vi "SteuerungWaermepumpe.vi"() -> ()   [LabVIEW 2015]
uses:
  <vilib>/DAQmx/read.llb/DAQmx Read.vi
  <vilib>/DAQmx/read.llb/DAQmx Read (Analog 1D Wfm NChan NSamp).vi
  <vilib>/DAQmx/write.llb/DAQmx Write.vi
  <vilib>/DAQmx/write.llb/DAQmx Write (Analog 1D Wfm NChan 1Samp).vi
  <vilib>/MakerHub/LINX/Public/Peripherals/Digital/Digital Write N Chans.vi
  <vilib>/DAQmx/miscellaneous.llb/DAQmx Fill In Error Info.vi
  <vilib>/Utility/file.llb/Read Delimited Spreadsheet (DBL).vi
  <vilib>/MakerHub/LINX/LMH-LINX.lvlib
panel:
  in  "reinitialize? (F) in":bool
  in  "reinitialize? (F)":bool
  out "ist an!":string
  in  "zusätzlicher Druck":dbl
  in  "PI05 SW":dbl format="%.2f"
  out "p_liq_mittel":dbl
  out "p_liq":dbl
  out "Schleifendauer":dbl format="%.5f"
  out "Mittelwert 2":dbl
  in  "Mittelwert 2":bool
  in  "Mittelwert?":bool
  out "Mittelwert":dbl
  in  "Boolean":bool
  out "xi_r":dbl
  in  "Regler Senke":bool
  in  "reinitialize?":bool
  in  "TI35 SW":dbl=43.0 format="%.2f"
  in  "Drehzahl Bestätigung":bool
  in  "Drehzahl SW":dbl=1000.0 min=500.0 max=3000.0 step=1.0 format="%#_4g"
  out "Check":dbl format="%#_13g"
  in  "Regler Hochdruck":bool
  in  "PID Regelung Pumpe":bool
  in  "SW TI39":dbl
  out "Array":bool[](array[boolean])
  in  "LEDs 2":bool[](array[boolean])
  in  "Regelung HK":bool
  in  "zu":bool
  in  "auf":bool
  out "FI_Oel":dbl
  in  "RV 33":dbl(slide) scale=-1.0..1.0
  in  "tag":string
  out "Pumpenwerte":dbl[](array[numeric]) format="%.2f"
  out "Speichert!":bool
  out "Historie":string
  in  "Kommentar":string
  out "refnum out":refnum<file>
  in  "Identität":string(combo)
  in  "Zeit X in Minuten":dbl(slide)=5.0 min=0.0 max=15.0 scale=5.0..15.0
  out "TI 21a Warnungen":dbl
  out "Leistung":dynamicdata(graph)
  out "TI 37":dbl
  in  "Programm stoppen!":bool
  out "%":sgl(slide) scale=0.0..100.0
  out "kalt":bool
  out "warm":bool
  out "?":T1(array[cluster]) {"?" format="%#.4g"; "Konzentration_reich" format="%#.4g"}
  in  "Mit EES vergleichen":bool
  in  "FI13 SW in l/min":dbl=3.0 min=3.0 max=12.0 step=0.10000000149011612
  out "COP_Oel":dbl
  out "Q-Oel kW":dbl format="%_4g"
  in  "Dateiname":string
  in  "Comment":bool
  in  "Speichern":bool caption="Aktivieren"
  out "ZU     Ventilstellung 33     AUF":dbl(slide) scale=0.0..100.0 scale format="%.2f"
  in  "Regelventil 34":dbl(slide) min=0.0 max=100.0 step=0.009999999776482582 scale=0.0..100.0
  in  "Matlab":bool
  in  "?":T2(tab)
  out "?":dynamicdata(graph)
  out "?":waveform(dbl)(graph)
  out "?":dynamicdata(graph)
  out "PI 12":dbl format="%.2f"
  out "PI 11":dbl format="%.2f"
  out "Dichte":dbl format="%.5g"
  in  "?":bool
  out "Betriebszeit":cluster{"second":i32, "minute":i32, "hour":i32}
  out "Temperatur Ölprüfstand":dbl
  out "FI 13 kg/min":dbl
  in  "Messung\nFrequenzwandler":bool
  out "Magnetventil":bool
  out "Fl.Pumpe an":bool
  out "Temperatur Öl":bool
  out "COP":dbl format="%#_13g"
  out "Verdichteraktivität":cluster{"second":i32, "minute":i32, "hour":i32}
  out "Q-Entgaser kW":dbl format="%_4g"
  out "Warnungen":bool[](array[boolean])
  out "Status Komponenten":bool[](array[boolean])
  in  "Sicherheits-Automatik":bool=TRUE
  out "Q-Resorber kW":dbl format="%_4g"
  out "Stellung Expansionsventil":waveform(dbl)(graph)
  out "FI 35 l/min":dbl format="%#_13g"
  out "FI 38 l/min":dbl format="%#_13g"
  out "FI Oel l/min":dbl format="%#.3g"
  out "LI in l":dbl format="%#_4g"
  out "TI 39":dbl format="%#_3g"
  out "TI 38":dbl format="%#_3g"
  out "TI 36":dbl format="%#_3g"
  out "TI 35":dbl format="%#_3g"
  out "TI 33":dbl format="%#_3g"
  out "TI 32":dbl format="%#_3g"
  out "TI 34":dbl format="%#_3g"
  out "TI 21a":dbl format="%#_3g"
  out "TI 21":dbl format="%#_3g"
  out "TI 20":dbl format="%#_3g"
  out "TI 14a":dbl format="%#_3g"
  out "TI 14":dbl format="%#_3g"
  out "TI 13":dbl format="%#_3g"
  out "TI 12":dbl format="%#_3g"
  out "TI 11":dbl format="%#_3g"
  out "TI 10":dbl format="%#_3g"
  out "TI 09":dbl format="%#_3g"
  out "TI 08":dbl format="%#_3g"
  out "TI 07":dbl format="%#_3g"
  out "TI 06a":dbl format="%#_3g"
  out "TI 06":dbl format="%#_3g"
  out "TI 05":dbl format="%#_3g"
  out "TI 04":dbl format="%#_3g"
  out "TI 22":dbl format="%#_3g"
  out "TI 02":dbl format="%#_3g"
  out "TI 01":dbl format="%#_3g"
  out "Konzentration":dbl format="%#_5g"
  in  "Pumpensteuerung":dbl min=0.0 max=10.0 step=0.009999999776482582 format="%.2g"
  out "PI 08":dbl format="%.2f"
  out "PI 05":dbl format="%#.2f"
  out "PI 02":dbl format="%.2f"
  out "PI 04":dbl format="%.2f"
  out "PDI 8-9":dbl format="%.2f"
  out "PI 14":dbl format="%.2f"
  out "PI 01":dbl format="%.2f"
  out "ZU    Ventilstellung Exp.V     AUF":dbl(slide) scale=0.0..100.0 scale format="%#.1f"
  in  "Exp.V":dbl(slide)=3.0 min=0.0 max=100.0 step=1.0 scale=0.0..100.0 scale format="%#.0f"
  out "ZU    Ventilstellung 14      AUF":dbl(slide) caption="Auf    Ventilstellung 14      Zu" scale=0.0..100.0 scale format="%#.2f"
  in  "Regelventil 36":dbl(slide) min=0.0 max=100.0 step=0.009999999776482582 scale=0.0..100.0 scale format="%#.0f"
  out "ZU  Ventilstellung 35  AUF":dbl(slide) scale=0.0..100.0 scale format="%.2f"
  in  "Regelventil 35":dbl(slide)=100.0 min=0.0 max=100.0 step=0.009999999776482582 scale=0.0..100.0 scale format="%#.3g"
  out "ZU     Ventilstellung 39     AUF":dbl(slide) scale=0.0..100.0 scale format="%.2f"
  in  "Regelventil 39":dbl(slide)=100.0 min=0.0 max=100.0 step=0.009999999776482582 scale=0.0..100.0
  out "Abscheider":cluster{dbl, dbl, dbl}(slide) scale=0.0..1.3
  out "FI 13 l/min":dbl format="%.2f"
  out "FI 07 l/min":dbl format="%.2f"
  out "LI in m":dbl format="%.2f"
  out "PDI 5-6":dbl format="%.4f"
  out "PI 07":dbl format="%.2f"
  out "Druckverhältnis":dbl
  out "Drehzahl":dbl
  out "Drehmoment":dbl
  out "Frequenz":dbl
  out "Leistung":dbl
  out "Durchfluss":waveform(dbl)[](graph)
  in  "Tab Control Temperaturen":T3(tab)
  out "Temperatur Reich":waveform(dbl)[](graph)
  out "Temperatur Arm":waveform(dbl)[](graph)
  out "Temperatur Öl":waveform(dbl)[](graph)
  out "Temperatur Senke/Quelle":waveform(dbl)[](graph)
  out "Druck":waveform(dbl)[](graph)
  # "Öltemperatur"
  # "Resorber"
  # "Entgaser"
  # "Druckverhältnis"
  # "ExpV"
  # "Verdichter an"
  # "iWÜ"
  # "Magnetventil"
  # "RV 39"
  # "RV 35"
  # "RV 33"
  # "RV 34"
  # "Pumpe an"
  # "Ölabscheider"
  # "2"
  # "1"
  # "RV 30"
  # "Verdichter"
  # "Pumpe"
  # "Leistung"
  # "kW"
  # "Speed"
  # "rpm"
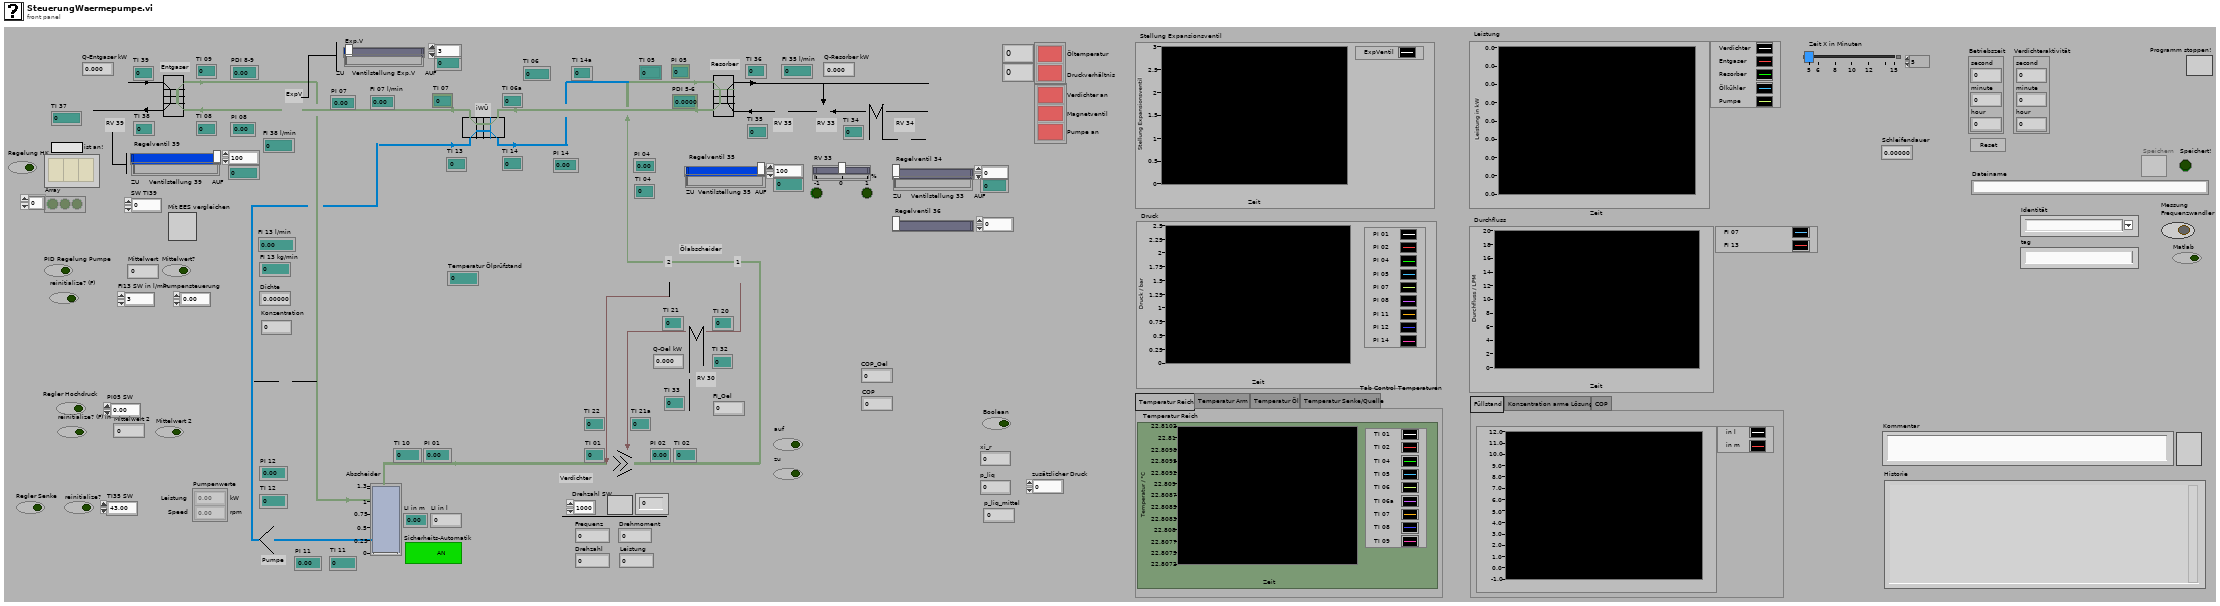
[diagram p1: front panel]
types:
  T1 = cluster{dbl, "Konzentration_reich":dbl, "String":string, bool}[]
  T2 = enum32{"Füllstand", "Konzentration arme Lösung", "COP"}
  T3 = enum32{"Temperatur Reich", "Temperatur Arm", "Temperatur Öl", "Temperatur Senke/Quelle"}
  T4 = enum8{"Enabled", "Disabled", "Disabled and Grayed Out"}
  T5 = typedef "LMH-LINX.lvlib/LINX Ref.ctl" = cluster{"Platform":T6, "Interface":T7, "LINX Device Config":T8}
  T6 = typedef "LMH-LINX.lvlib/Platform.ctl" = enum16{"LINX", "myRIO"}
  T7 = typedef "LMH-LINX.lvlib/Interface.ctl" = enum16{"Serial", "TCP"}
  T8 = typedef "LMH-LINX.lvlib/Device.lvlib/LINX Device Config.ctl" = cluster{"Interface":T7, "COM Port":refnum<visa-resource-name>, "TCP Configuration":T9, "Device Family":u8, "Device ID":u8, "Device Name":string, "TCP Ref":refnum<k5>, "Channels":T10}
  T9 = typedef "LMH-LINX.lvlib/Device.lvlib/TCP Config.ctl" = cluster{"IP Address":string, "Port":u16}
  T10 = typedef "LMH-LINX.lvlib/Channels.ctl" = cluster{"DI":u8[], "DO":u8[], "AI":u8[], "AO":u8[], "PWM":u8[], "QE":u8[], "UART":u8[], "I2C 2":u8[], "SPI":u8[], "CAN":u8[], "Servo":u8[], "AI Ref (V)":dbl, "AO Ref (V)":dbl, "AO Resolution (Bits)":u8}
  T11 = enum16{"open", "replace", "create", "open or create", "replace or create", "replace or create with confirmation"}
  T12 = cluster{"Array[0]":dbl, "Array[1]":dbl, "Array[2]":dbl}
  T13 = cluster{"Array[0]":sgl, "Array[1]":sgl, "Array[2]":sgl}
  T14 = cluster{"Numeric":dbl, "Konzentration_reich":sgl, "String":string, bool}[]
  T15 = typedef "LVDateTimeRec.ctl" = cluster{"fractional second":dbl, "second":i32, "minute":i32, "hour":i32, "day of month":i32, "month":i32, "year":i32, "day of week":i32, "day of year":i32, "DST":i32}
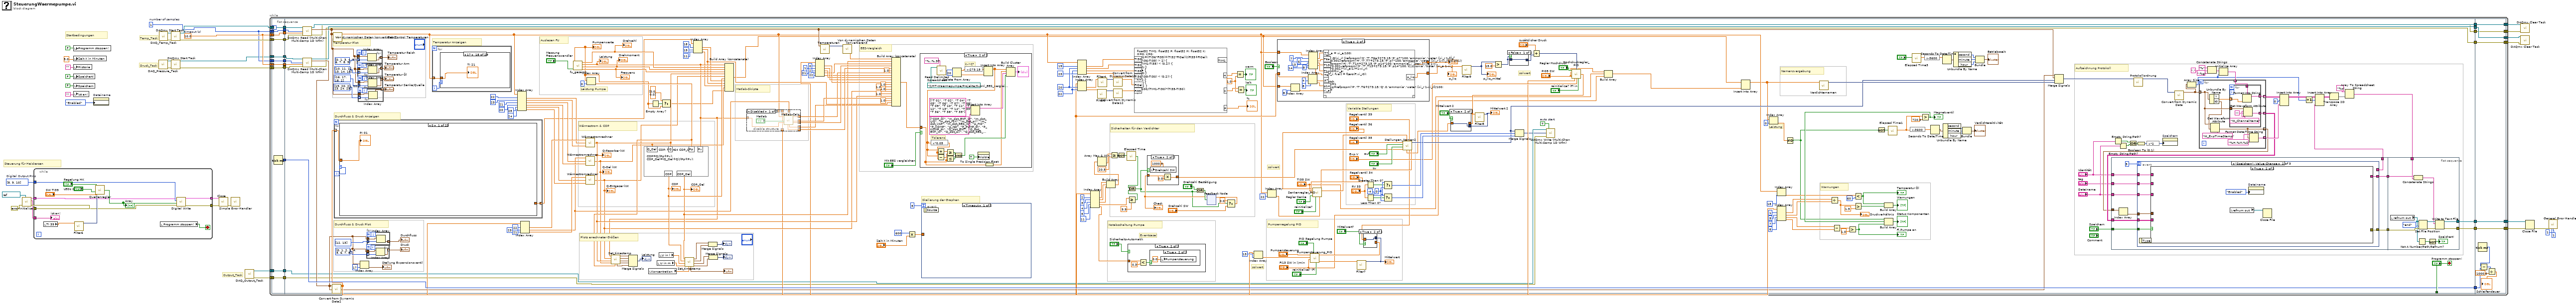
[diagram p0: block diagram]
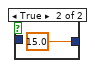
[diagram p3: hidden frame]
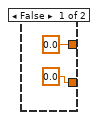
[diagram p6: hidden frame]
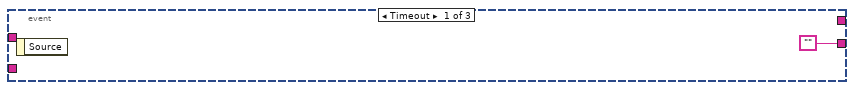
[diagram p8: hidden frame]
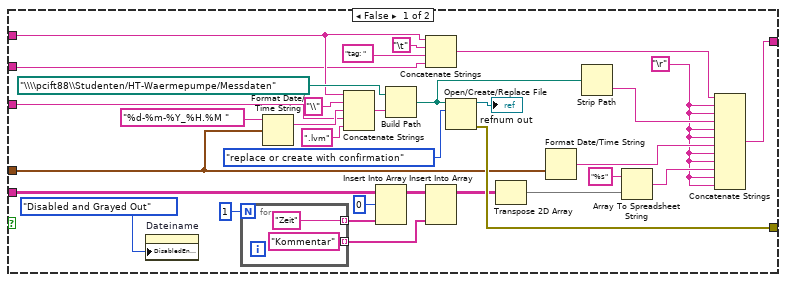
[diagram p9: hidden frame]
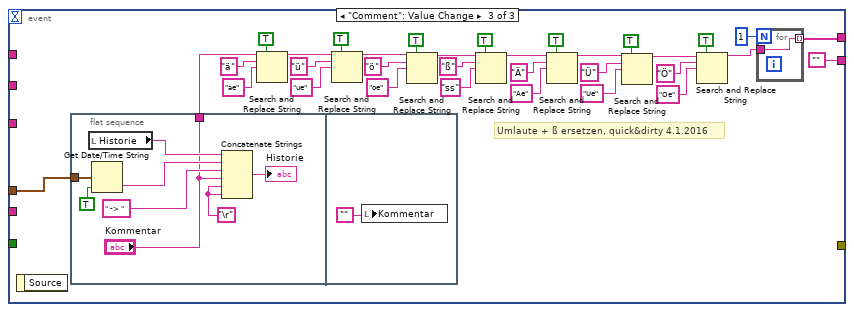
[diagram p10: hidden frame]
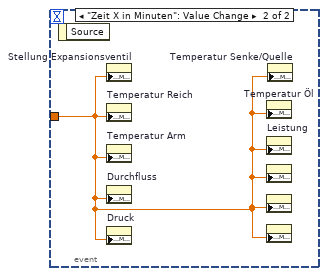
[diagram p11: hidden frame]
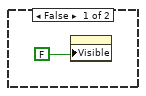
[diagram p12: hidden frame]
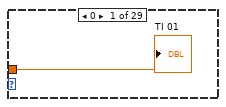
[diagram p15: hidden frame]
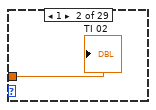
[diagram p16: hidden frame]
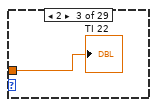
[diagram p17: hidden frame]
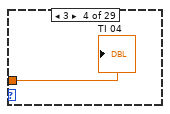
[diagram p18: hidden frame]
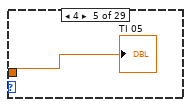
[diagram p19: hidden frame]
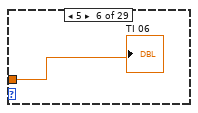
[diagram p20: hidden frame]
diagram:
  w9 = 10.0  # timeout (s)
  w8 = 1  # number of samples
  w21 = i32[] [8, 9, 10]  # Digital Output PIns
  # "Output_Task"
  # "Druck_Task"
  # "Temp_Task"
  # "Steuerung für Heizkerzen"
  # "Startbedingungen"
  n1 = call <vilib>:"Initialize.vi"("Serial Port"=refnum<visa-resource-name> "COM3", "Error In"=errorcluster {"status"=FALSE, "code"=0, "source"=""}) -> ("Error Out"=w22:errorcluster, "Device Name"=w19:string, "LINX Ref"=w25:T5)  [unwired: 7 in]
  n2 = while {
    tunnel: w25 -> [w40]
    tunnel: [w50] -> w24
    tunnel: [w49] -> w23
    tunnel: w22 -> [w39]
    tunnel: w21 -> [w48]
    tunnel: w19 -> [w38]
    stop <- w47 stop-if-true
    n3 = local read "TI 39"() -> (w41:dbl)
    n4 = call "Filter6"("Signal"=w41) -> ("Filtered Signal"=w42:dynamicdata)  [unwired: 9 in, 1 out]
    n5 = call "Quellenregler.vi"("Regelung Quelle"="Regelung HK", "TI 38 IW °C"=w42, "LEDs"="LEDs 2", "TI 38 SW °C"="SW TI39") -> ("Kerzen von Regler"=w44:bool[])  [unwired: 3 in, 1 out]
    "Array" <- w44
    n6 = local read "Programm stoppen!"() -> (w47:bool)
    n7 = call-poly <vilib>:"Digital Write.vi"("Error In"=w39, "Values"=w44, "DO Channels"=w48, "LINX Resource"=w40) -> ("Error Out"=w49:errorcluster, "LINX Resource"=w50:T5)  [unwired: 6 in]
    "ist an!" <- w38
  }
  n8 = local write "Programm stoppen!"(FALSE ("Programm stoppen!")) -> ()
  n9 = local write "Zeit X in Minuten"(5.0 ("Zeit X in Minuten")) -> ()
  n10 = local write "Historie"("") -> ()
  n11 = local write "Speichert!"(FALSE ("Speichert!")) -> ()
  n12 = local write "Speichern"(FALSE ("Speichern")) -> ()
  n13 = local write "ist an!"("") -> ()
  n14 = property on="Dateiname" class="Str"("DisabledEnum"=T4."Enabled" ("Disabled")) -> ()  [unwired: 2 in, 2 out]
  n15 = call "DAQ_Pressure_Task.vi"() -> ("error out"=w13:errorcluster, "task out"=w14:refnum<k21>)  [unwired: 10 in]
  n16 = call "DAQ_Temp_Task.vi"() -> ("error out"=w15:errorcluster, "task out"=w16:refnum<k21>)  [unwired: 10 in]
  n17 = call <vilib>:"DAQmx Start Task.vi"("task/channels in"=w14, "error in"=w13) -> ("task out"=w7:refnum<k21>, "error out"=w10:errorcluster)  [unwired: 12 in]
  n18 = call <vilib>:"DAQmx Start Task.vi"("task/channels in"=w16, "error in"=w15) -> ("task out"=w11:refnum<k21>, "error out"=w12:errorcluster)  [unwired: 12 in]
  n19 = call <vilib>:"Close.vi"("Error In"=w23, "LINX Resource"=w24) -> ("Error Out"=w26:errorcluster)  [unwired: 8 in, 1 out]
  n20 = call <vilib>:"Simple Error Handler.vi"("error in (no error)"=w26) -> ()  [unwired: 4 in, 5 out]
  n21 = call "DAQ_Output_Task.vi"() -> ("error out"=w1:errorcluster, "task out"=w2:refnum<k21>)  [unwired: 10 in]
  n22 = while {
    tunnel: [w85] -> w31
    tunnel: [w84] -> w30
    tunnel: w12 -> [w78]
    tunnel: w9 -> [w76]
    tunnel: w11 -> [w73]
    tunnel: w8 -> [w71]
    tunnel: w10 -> [w69]
    tunnel: w9 -> [w68]
    tunnel: w8 -> [w66]
    tunnel: w7 -> [w64]
    tunnel: [w60] -> w6
    tunnel: [w59] -> w5
    tunnel: [w57] -> w4
    tunnel: [w55] -> w3
    tunnel: w2 -> [w54]
    tunnel: w1 -> [w51]
    stop <- w83 stop-if-true
    n23 = flat-sequence {
      tunnel: [w96] -> w79
      tunnel: w78 -> [w95]
      tunnel: [w95] -> w77
      tunnel: w76 -> [w94]
      tunnel: [w94] -> w75
      tunnel: w73 -> [w93]
      tunnel: [w93] -> w74
      tunnel: [w92] -> w72
      tunnel: w71 -> [w92]
      tunnel: [w91] -> w70
      tunnel: w69 -> [w91]
      tunnel: w68 -> [w90]
      tunnel: [w90] -> w67
      tunnel: w66 -> [w89]
      tunnel: [w89] -> w65
      tunnel: w64 -> [w88]
      tunnel: [w88] -> w63
      tunnel: w54 -> [w87]
      tunnel: [w87] -> w53
      tunnel: [w86] -> w52
      tunnel: w51 -> [w86]
      tunnel: ["Programm stoppen!"] -> w83
      tunnel: [w294] -> w82
      tunnel: [w293] -> w81
      tunnel: [w176] -> w80
      tunnel: w79 -> [w176]
      tunnel: w77 -> [w126]
      tunnel: w75 -> [w125]
      tunnel: w74 -> [w124]
      tunnel: w72 -> [w123]
      tunnel: w70 -> [w122]
      tunnel: w67 -> [w121]
      tunnel: w65 -> [w120]
      tunnel: w63 -> [w119]
      tunnel: [w118] -> w62
      tunnel: [w117] -> w61
      tunnel: [w116] -> w58
      tunnel: [w115] -> w56
      tunnel: w53 -> [w113]
      tunnel: w52 -> [w112]
      tunnel: [w703] -> w84
      tunnel: [w704] -> w85
      tunnel: w82 -> [w704]
      tunnel: w81 -> [w703]
      tunnel: w80 -> [w701]
      tunnel: w62 -> [w696]
      tunnel: w61 -> [w697]
      tunnel: [w697] -> w60
      tunnel: [w696] -> w59
      tunnel: w58 -> [w695]
      tunnel: [w695] -> w57
      tunnel: w56 -> [w694]
      tunnel: [w694] -> w55
      frame #0 {
        n24 = Tick Count (ms)() -> (millisecond timer value=w96:u32)
      }
      frame #1 {
        w114 = TRUE  # auto start
        w314 = sgl 1.0
        w327 = 22
        w332 = 20
        w358 = -4
        w359 = 0
        # "solwert"
        # "solwert"
        # "solwert"
        # "Sicherheiten für den Verdichter"
        # "Pumpenregelung PID"
        # "Skalierung der Graphen"
        # "Leistung Pumpe"
        # "Leistung"
        # "Eventcase!"
        # "Durchfluss & Druck Anzeigen"
        # "Temperatur Anzeigen"
        # "Plots errechneter Größen"
        # "EES-Vergleich"
        # "Matlab-Skripte"
        # "Warnungen"
        # "Namensvergebung"
        # "Wärmestrom & COP"
        # "Notabschaltung Pumpe"
        # "Auslesen FU"
        # "Durchfluss & Druck Plot"
        # "Temperatur Plot"
        # "Aufzeichnung Protokoll"
        # "Variable Stellungen"
        n25 = call-poly "DAQmx Read (Multi-Chan Multi-Samp 1D Wfm).vi"("task/channels in"=w124, "number of samples per channel"=w123, "timeout"=w125, "error in"=w126) -> ("task out"=w117:refnum<k21>, "data"=w127:waveform(dbl)[], "error out"=w116:errorcluster)  [unwired: 9 in]
        n26 = call-poly "DAQmx Read (Multi-Chan Multi-Samp 1D Wfm).vi"("task/channels in"=w119, "number of samples per channel"=w120, "timeout"=w121, "error in"=w122) -> ("task out"=w118:refnum<k21>, "data"=w128:waveform(dbl)[], "error out"=w115:errorcluster)  [unwired: 9 in]
        n27 = call "Convert from Dynamic Data2"("Dynamic Data Type"=w128) -> ("Array"=w133:dbl[])  [unwired: 3 in]
        n28 = call "Von dynamischen Daten konvertieren2"("Dynamic Data Type"=w127) -> ("Array"=w108:dbl[])  [unwired: 3 in]
        n29 = for {
          tunnel: w133 -> [w642] mode=indexing
          tunnel: [w641] -> w138 mode=indexing
          i -> [w643]
          n30 = case shown="0" w643 {
            tunnel: w642 -> [w644 w645 w646 w647 w648 w649 w650 w651 w652 w653 w654 w663 w675 w678 w679 w680 w681 w682 w685 w689 w690 w691 w692 w693 _]
            tunnel: [_ _ _ _ _ _ _ _ _ _ _ w655 _ _ _ _ _ _ w683 w687 _ _ _ _ _] -> w641
            frame 0 {
              "PI 01" <- w644
            }
            frame 1 {
              "PI 02" <- w645
            }
            frame 2 {
              "PI 04" <- w646
            }
            frame 3 {
              "PI 05" <- w647
            }
            frame 4 {
              "PI 07" <- w648
            }
            frame 5 {
              "PI 08" <- w649
            }
            frame 6 {
              "PI 11" <- w650
            }
            frame 7 {
              "PI 12" <- w651
            }
            frame 8 {
              "PI 14" <- w652
            }
            frame 9 {
              "PDI 5-6" <- w653
            }
            frame 10 {
              "PDI 8-9" <- w654
            }
            frame 11 {
              n31 = call "Filter3"("Signal"=w663) -> ("Filtered Signal"=w661:dynamicdata)  [unwired: 9 in, 1 out]
              n32 = Greater?(x=w663, y=0.3) -> (0:w658:bool)
              n33 = case shown="False" w658 {
                tunnel: w663 -> [_ w674]
                tunnel: [0.0 w674] -> w666
                frame False {
                }
                frame True {
                }
              }
              n34 = call "Convert from Dynamic Data6"("Dynamic Data Type"=w661) -> ("Scalar"=w660:dbl)  [unwired: 3 in]
              n35 = Multiply(x=w660, y=10.0) -> (x*y=w662:dbl)
              n36 = Greater?(x=w663, y=0.4) -> (0:w659:bool)
              n37 = formula code="float64 y; float64 Vu; /*Vu: Volumen schmaler Zylinder+Fuellstandsmesser*/\nVu=10;  /* 10 Liter */\n\nif (x<=10.25) \ny=(x-1)*pi*(0.536**2+0.32**2);\nelse\ny=Vu+(x-10.25)*pi*(1.584**2+0.32**2);"("x"=w662) -> ("y"=w655:dbl)
              "LI in l" <- w655
              n38 = case shown="False" w659 {
                tunnel: w663 -> [_ w672]
                tunnel: [0.0 w672] -> w665
                frame False {
                }
                frame True {
                }
              }
              n39 = Merge Signals(w663, w666, w665) -> (w667:dynamicdata)
              n40 = call "Convert from Dynamic Data3"("Dynamic Data Type"=w667) -> ("Array"=w670:dbl[])  [unwired: 3 in]
              n41 = Array To Cluster(array=w670) -> (cluster=w657:T12)
              n42 = To Single Precision Float(number=w657) -> (single precision float=→"Abscheider":T13)
              "LI in m" <- w663
            }
            frame 12 {
              "FI 07 l/min" <- w675
            }
            frame 13 {
              n43 = local read "Dichte"() -> (w677:dbl)
              n44 = Multiply(x=w678, y=w677) -> (x*y=→"FI 13 kg/min":dbl)
              "FI 13 l/min" <- w678
            }
            frame 14 {
              "ZU     Ventilstellung 39     AUF" <- w679
              "ZU     Ventilstellung 33     AUF" <- w679
            }
            frame 15 {
              "ZU  Ventilstellung 35  AUF" <- w680
            }
            frame 16 {
              # "RV14 ist entfernt"
              "ZU    Ventilstellung 14      AUF" <- w681
            }
            frame 17 {
              "ZU    Ventilstellung Exp.V     AUF" <- w682
            }
            frame 18 {
              n45 = call "Filter"("Signal"=w685) -> ("Filtered Signal"=w684:dynamicdata)  [unwired: 9 in, 1 out]
              n46 = call "Convert from Dynamic Data4"("Dynamic Data Type"=w684) -> ("Scalar"=w686:dbl)  [unwired: 3 in]
              n47 = formula code="float64 D;\nD=9.375*StromDichte+0.7125;\nD=floor(D*100000)/100000;"("StromDichte"=w686) -> ("D"=w683:dbl)
              "Dichte" <- w683
            }
            frame 19 {
              n48 = call "Filter2"("Signal"=w689) -> ("Filtered Signal"=w688:dynamicdata)  [unwired: 9 in, 1 out]
              n49 = To Double Precision Float(number=w688) -> (double precision float=w687:dbl)
              "Konzentration" <- w687
            }
            frame 20 {
              "FI Oel l/min" <- w690
            }
            frame 21 {
              "FI 38 l/min" <- w691
            }
            frame 22 {
              "FI 35 l/min" <- w692
            }
            frame 23 {
              "FI_Oel" <- w693
            }
            frame 24, Default {
            }
          }
        }
        n50 = for {
          tunnel: i32[] [0, 1, 3, 4, 5, 6, 7, 8, 9] -> [w455] mode=indexing
          tunnel: w127 -> [w454]
          tunnel: [w453] -> w230 mode=indexing
          n51 = Index Array(array=w454, index=w455) -> (element=w453:waveform(dbl))
        }
        "Temperatur Reich" <- w230
        n52 = for {
          tunnel: i32[] [10, 11, 12, 13, 14, 15] -> [w452] mode=indexing
          tunnel: w127 -> [w451]
          tunnel: [w450] -> w231 mode=indexing
          n53 = Index Array(array=w451, index=w452) -> (element=w450:waveform(dbl))
        }
        "Temperatur Arm" <- w231
        n54 = for {
          tunnel: i32[] [16, 17, 18, 2] -> [w449] mode=indexing
          tunnel: w127 -> [w448]
          tunnel: [w447] -> w232 mode=indexing
          n55 = Index Array(array=w448, index=w449) -> (element=w447:waveform(dbl))
        }
        "Temperatur Öl" <- w232
        n56 = for {
          tunnel: i32[] [19, 20, 21, 22, 23, 24, 25] -> [w446] mode=indexing
          tunnel: w127 -> [w445]
          tunnel: [w444] -> w233 mode=indexing
          n57 = Index Array(array=w445, index=w446) -> (element=w444:waveform(dbl))
        }
        "Temperatur Senke/Quelle" <- w233
        n58 = Index Array(array=w128, index=17) -> (element=→"Stellung Expansionsventil":waveform(dbl))
        n59 = for {
          tunnel: [w440] -> w228 mode=indexing
          tunnel: w128 -> [w439]
          tunnel: i32[] [0, 1, 2, 3, 4, 5, 6, 7, 8] -> [w438] mode=indexing
          n60 = Index Array(array=w439, index=w438) -> (element=w440:waveform(dbl))
        }
        "Druck" <- w228
        n61 = for {
          tunnel: [w443] -> w229 mode=indexing
          tunnel: w128 -> [w442]
          tunnel: i32[] [12, 13] -> [w441] mode=indexing
          n62 = Index Array(array=w442, index=w441) -> (element=w443:waveform(dbl))
        }
        "Durchfluss" <- w229
        n63 = for {
          tunnel: w108 -> [w611] mode=indexing
          i -> [w612]
          n64 = case shown="17" w612 {
            tunnel: w611 -> [w613 w614 w615 w616 w617 w618 w619 w620 w621 w622 w623 w624 w625 w626 w627 w628 w629 w630 w631 w632 w633 w634 w635 w636 w637 w638 w639 w640 _]
            frame 0 {
              "TI 01" <- w613
            }
            frame 1 {
              "TI 02" <- w614
            }
            frame 2 {
              "TI 22" <- w615
            }
            frame 3 {
              "TI 04" <- w616
            }
            frame 4 {
              "TI 05" <- w617
            }
            frame 5 {
              "TI 06" <- w618
            }
            frame 6 {
              "TI 06a" <- w619
            }
            frame 7 {
              "TI 07" <- w620
            }
            frame 8 {
              "TI 08" <- w621
            }
            frame 9 {
              "TI 09" <- w622
            }
            frame 10 {
              "TI 10" <- w623
            }
            frame 11 {
              "TI 11" <- w624
            }
            frame 12 {
              "TI 12" <- w625
            }
            frame 13 {
              "TI 13" <- w626
            }
            frame 14 {
              "TI 14" <- w627
            }
            frame 15 {
              "TI 14a" <- w628
            }
            frame 16 {
              "TI 20" <- w629
            }
            frame 17 {
              "TI 21" <- w630
            }
            frame 18 {
              "TI 21a" <- w631
              "TI 21a Warnungen" <- w631
            }
            frame 19 {
              # "Check T_Heater"
              "TI 34" <- w632
            }
            frame 20 {
              "TI 32" <- w633
            }
            frame 21 {
              "TI 33" <- w634
            }
            frame 22 {
              "TI 35" <- w635
            }
            frame 23 {
              "TI 36" <- w636
            }
            frame 24 {
              "TI 38" <- w637
            }
            frame 25 {
              "TI 39" <- w638
            }
            frame 26 {
              "Temperatur Ölprüfstand" <- w639
            }
            frame 27 {
              "TI 37" <- w640
            }
            frame 28, Default {
            }
          }
        }
        n65 = Index Array(array=w108, index #1=22 ("index"), index #2=23 ("index"), index #3=21 ("index"), index #4=20 ("index"), index #5=25 ("index"), index #6=24 ("index")) -> (element #1=w261:dbl, element #2=w260:dbl, element #3=w259:dbl, element #4=w258:dbl, element #5=w257:dbl, element #6=w256:dbl)
        n66 = Index Array(array=w133, index #1=22 ("index"), index #2=23 ("index"), index #3=21 ("index")) -> (element #1=w263:dbl, element #2=w239:dbl, element #3=w262:dbl)
        n67 = call "fu_gesamt.vi"("Boolean"="Messung\nFrequenzwandler") -> ("Frequenz"=w251:dbl, "Drehmoment"=w252:dbl, "Leistung"=w152:dbl, "Drehzahl"=w253:dbl, "Scaled"=w98:dbl[])  [unwired: 6 in]
        "Leistung" <- w152
        "Frequenz" <- w251
        "Drehmoment" <- w252
        "Drehzahl" <- w253
        "Pumpenwerte" <- w98
        n68 = call "Wärmestromrechner.vi"("Taus"=w260, "Tein"=w261, "Massenstrom"=w263) -> ("Wärmestrom Q"=w153:dbl)  [unwired: 2 in]
        "Q-Resorber kW" <- w153
        n69 = call "Wärmestromrechner.vi"("Taus"=w258, "Tein"=w259, "Massenstrom"=w239) -> ("Wärmestrom Q"=w139:dbl)  [unwired: 2 in]
        "Q-Oel kW" <- w139
        n70 = call "Wärmestromrechner.vi"("Taus"=w256, "Tein"=w257, "Massenstrom"=w262) -> ("Wärmestrom Q"=w151:dbl)  [unwired: 2 in]
        "Q-Entgaser kW" <- w151
        n71 = Index Array(array=w98, index=0) -> (element=w154:dbl)
        n72 = call "Set_timestamp.vi"("Eingang 5"=w154, "Eingang 4"=w139, "Eingang 3"=w153, "Eingang 2"=w151, "Eingang"=w152) -> ("Ausgang 4"=w149:waveform(dbl), "Ausgang 3"=w148:waveform(dbl), "Ausgang 2"=w147:waveform(dbl), "Ausgang"=w146:waveform(dbl), "Ausgang 5"=w150:waveform(dbl))  [unwired: 2 in]
        n73 = Merge Signals(w146, w147, w148, w149, w150) -> (→"Leistung":dynamicdata)
        n74 = formula code="float64 COP; float64 COP_Oel;\n\nCOP=Q/(Pp+Pv);\nCOP_Oel=(Q_Oel+Q)/(Pp+Pv);"("Pv"=w152, "Q"=w153, "Pp"=w154, "Q_Oel"=w139) -> ("COP"=w162:dbl, "COP_Oel"=w161:dbl)
        "COP" <- w162
        "COP_Oel" <- w161
        n75 = local read "Konzentration"() -> (w166:dbl)
        n76 = Empty Array?(array=w98) -> (empty?=w100:bool)
        n77 = local read "LI in m"() -> (w164:dbl)
        n78 = local read "LI in l"() -> (w163:dbl)
        n79 = Select(t=dbl[] [0.0, 0.0], s=w100, f=w98) -> (s? t:f=w97:dbl[])
        n80 = call "Set_timestamp.vi"("Eingang 5"=w166, "Eingang 4"=w164, "Eingang 3"=w163, "Eingang 2"=w162, "Eingang"=w161) -> ("Ausgang 4"=w159:waveform(dbl), "Ausgang 3"=w158:waveform(dbl), "Ausgang 2"=w156:waveform(dbl), "Ausgang"=w155:waveform(dbl), "Ausgang 5"=→"?":waveform(dbl))  [unwired: 2 in]
        n81 = Index Array(array=w138, index #1=18 ("index"), index #2=19 ("index"), index #3=11 ("index")) -> (element #1=w140:dbl, element #2=w137:dbl, element #3=w141:dbl)
        n82 = Merge Signals(w155, w156) -> (→"?":dynamicdata)
        n83 = Merge Signals(w158, w159) -> (→"?":dynamicdata)
        n84 = Build Array (concatenate)(w152, w253, w252, w251, w153, w151, w162, w140, w137, w141, w139, w97) -> (w103:dbl[])
        n85 = disable-structure shown="Disabled" {
          disable-tunnel: [w401 _] -> w355
          disable-tunnel: [w400 _] -> w344
          disable-tunnel: [w399 _] -> w333
          disable-tunnel: [w398 _] -> w255
          disable-tunnel: [w397 _] -> w250
          disable-tunnel: w239 -> [w396 _]
          disable-tunnel: w152 -> [w395 _]
          disable-tunnel: w133 -> [w394 w403]
          disable-tunnel: w108 -> [w393 _]
          disable-tunnel: [_ w403] -> _
          frame Disabled {
            n86 = call "Matlab-Calc.vi"("Temp-Array"=w393, "Matlab?"="Matlab", "Leistung"=w395, "Druck-Array"=w394, "FI Öl"=w396) -> ("m_reich [g/s]"=w400:dbl, "Konzentration_reich"=w397:dbl, "m_arm [g/s]"=w401:dbl, "Dampfmassenstrom [g/s]"=w398:dbl, "Dampfmassenanteil"=w399:dbl)  [unwired: 3 in, 7 out]
          }
          frame Enabled {
          }
        }
        n87 = Index Array(array=w133, index #1=0 ("index"), index #2=1 ("index"), index #3=2 ("index"), index #4=21 ("index"), index #5=22 ("index")) -> (element #1=w338:dbl, element #2=w339:dbl, element #3=w340:dbl, element #4=w337:dbl, element #5=w335:dbl)
        n88 = call "Temperaturen"("Signals"=w127) -> ("Signal Out"=w345:dynamicdata)  [unwired: 9 in, 1 out]
        n89 = call "Von dynamischen Daten konvertieren3"("Dynamic Data Type"=w345) -> ("Array"=w346:dbl[])  [unwired: 3 in]
        n90 = Build Array (concatenate)(w346, w161, w337, w355, w344, 1.0 ("element"), w255, w335, w340, w339, w338, 1.0 ("element"), 1.0 ("element"), 1.0 ("element"), w151, 1.0 ("element"), w153, w333, 1.0 ("element"), w137, w250) -> (w347:dbl[])
        n91 = Multiply(x=600, y="Zeit X in Minuten") -> (x*y=w306:dbl)
        n92 = case shown="True" "Mit EES vergleichen" {
          tunnel: w347 -> [_ w589]
          frame False {
            n93 = property class="Arr (strict)"("Visible"=FALSE) -> ()  [unwired: 2 in, 2 out]
          }
          frame True {
            # "K->C°"
            # "Toleranz"
            n94 = call-poly <vilib>:"Read Delimited Spreadsheet.vi"("file path (dialog if empty)"=path "Z:/HT-Waermepumpe/Projekte/SubVi_EES_vergleich/test.txt", "format (%.3f)"="%,;%.3f") -> ("first row"=w594:dbl[])  [unwired: 8 in, 5 out]
            n95 = Delete From Array(array=w594, length=20) -> (deleted portion=w590:dbl[], array with subset deleted=w592:dbl[])  [unwired: 1 in]
            n96 = expression code="x-273.15"(w592) -> (w591:dbl[])
            n97 = Insert Into Array(array=string[] ["T 01", "T 02", "T 04", "T 05", "T 06", "T 07", "T 08", "T 09", "T 10", "T 11", "T 12", "T 13", "T 14", "T 35", "T 36", "T 38", "T 39"] ("Array"), new element=string[] ["COP_Öl", "m_dot_ENT_W", "m_dot_LIQ", "m_dot_MIX", "m_dot_oil", "m_dot_VAP", "m_dot_RES_W", "p_HD", "P_KOMP", "p_ND", "P_PUMP_th", "P_KOMP_th", "Q_dot_ENT", "Q_dot_ENT_W", "Q_dot_oil", "Q_dot_RES_W", "q_geg", "Q_dot_RES", "xi_LIQ", "xi_MIX"] ("Array")) -> (w601:string[])  [unwired: 1 in]
            n98 = property class="Arr (strict)"("Visible"=TRUE) -> ()  [unwired: 2 in, 2 out]
            n99 = Insert Into Array(array=w591, new element=w590) -> (w586:dbl[])  [unwired: 1 in]
            n100 = expression code="x*0.05"(w586) -> (w588:dbl[])
            n101 = Add(x=w586, y=w588) -> (x+y=w597:dbl[])
            n102 = Subtract(x=w586, y=w588) -> (x-y=w596:dbl[])
            n103 = Greater Or Equal?(x=w597, y=w589) -> (x >= y?=w598:bool[])
            n104 = Less Or Equal?(x=w596, y=w589) -> (x <= y?=w599:bool[])
            n105 = And(x=w598, y=w599) -> (x .and. y?=w595:bool[])
            n106 = To Single Precision Float(number=w589) -> (single precision float=w587:sgl[])
            n107 = Build Cluster Array(w586, w587, w601, w595) -> (→"?":T14)
          }
        }
        n108 = event shown="[0] Timeout" {
          selector: _ -> [_ _]
          dyn-events: _ -> [_ _]
          timeout: 5 -> [_ _]
          tunnel: w306 -> [_ w584]
          event Timeout {
            n109 = event-data() -> ()  [unwired: 1 in, 1 out]
          }
          event "Zeit X in Minuten": Value Change {
            n110 = event-data() -> ()  [unwired: 1 in, 1 out]
            n111 = property on="Stellung Expansionsventil" class="WFChart (strict)"("XScale.Maximum"=w584) -> ()  [unwired: 2 in, 2 out]
            n112 = property on="Temperatur Reich" class="WFChart (strict)"("XScale.Maximum"=w584) -> ()  [unwired: 2 in, 2 out]
            n113 = property on="Temperatur Arm" class="WFChart (strict)"("XScale.Maximum"=w584) -> ()  [unwired: 2 in, 2 out]
            n114 = property on="Durchfluss" class="WFChart (strict)"("XScale.Maximum"=w584) -> ()  [unwired: 2 in, 2 out]
            n115 = property on="Druck" class="WFChart (strict)"("XScale.Maximum"=w584) -> ()  [unwired: 2 in, 2 out]
            n116 = property on="Temperatur Öl" class="WFChart (strict)"("XScale.Maximum"=w584) -> ()  [unwired: 2 in, 2 out]
            n117 = property on="Leistung" class="WFChart (strict)"("XScale.Maximum"=w584) -> ()  [unwired: 2 in, 2 out]
            n118 = property class="WFChart (strict)"("XScale.Maximum"=w584) -> ()  [unwired: 2 in, 2 out]
            n119 = property class="WFChart (strict)"("XScale.Maximum"=w584) -> ()  [unwired: 2 in, 2 out]
            n120 = property class="WFChart (strict)"("XScale.Maximum"=w584) -> ()  [unwired: 2 in, 2 out]
            n121 = property on="Temperatur Senke/Quelle" class="WFChart (strict)"("XScale.Maximum"=w584) -> ()  [unwired: 2 in, 2 out]
          }
        }
        n122 = Index Array(array=w108, index #1=19, index #2=w332, index #3=w327, index #4=23) -> (element #1=w324:dbl, element #2=w323:dbl, element #3=w322:dbl, element #4=w321:dbl)
        n123 = Index Array(array=w133, index #1=w332, index #2=w327) -> (element #1=w330:dbl, element #2=w329:dbl)
        n124 = Index Array(array=w133, index #1=2 ("index"), index #2=3 ("index"), index #3=4, index #4=5, index #5=11 ("index")) -> (element #1=w209:dbl, element #2=w208:dbl, element #3=w207:dbl, element #4=w213:dbl, element #5=w184:dbl)
        n125 = call "Filter5"("Signal"=w329) -> ("Filtered Signal"=w325:dynamicdata)  [unwired: 9 in, 1 out]
        n126 = call "Filter4"("Signal"=w330) -> ("Filtered Signal"=w326:dynamicdata)  [unwired: 9 in, 1 out]
        n127 = Build Array(w209, w208, w207) -> (w206:dbl[])
        n128 = Array Max & Min(array=w206) -> (min value=w202:dbl)  [unwired: 3 out]
        n129 = Greater Or Equal?(x=w202, y=20.5 ("x")) -> (x >= y?=w205:bool)
        n130 = call "Convert from Dynamic Data11"("Dynamic Data Type"=w326) -> ("Scalar"=w320:dbl)  [unwired: 3 in]
        n131 = call "Convert from Dynamic Data12"("Dynamic Data Type"=w325) -> ("Scalar"=w319:dbl)  [unwired: 3 in]
        n132 = Not(x=w205) -> (.not. x?=w204:bool)
        n133 = call "Elapsed Time"("Reset"=w204) -> ("Time has Elapsed"=w203:bool)  [unwired: 11 in, 7 out]
        n134 = Greater Or Equal?(x=w213, y=9.9 ("x")) -> (x >= y?=w217:bool)
        n135 = case shown="True" "Sicherheits-Automatik" {
          tunnel: w184 -> [_ w608]
          frame False {
          }
          frame True {
            n136 = Less?(x=w608, y=0.3) -> (x < y?=w607:bool)
            n137 = case shown="True" w607 {
              frame False {
              }
              frame True {
                n138 = local write "Pumpensteuerung"(0.0) -> ()
              }
            }
          }
        }
        n139 = Or(x=w203, y=w217) -> (x .or. y?=w195:bool)
        n140 = formula code="float32 TIM1; float32 P; float32 H; float32 K;\nH=0; K=0;\nTIM1=((TI36*FI35)+(TI32*FIOel))/(FI35+FIOel);\nif((TI36-TI35) > 2) {\nif((TIM1-TI35) < (0.2)) {\nH=1;}\nelse {\nH=0;}\nif((TI35-TI30) < (0.2)) {\nK=1;}\nelse {\nK=0; }\nP=100/(TIM1-TI30)*(TI35-TI30);\n}"("TI30"=w324, "TI32"=w323, "TI35"=w322, "TI36"=w321, "FIOel"=w320, "FI35"=w319) -> ("H"=w318:sgl, "K"=w315:sgl, "P"=→"%":sgl)  [unwired: 1 out]
        n141 = Or(x="Drehzahl Bestätigung", y=w195) -> (x .or. y?=w197:bool)
        n142 = feedback #1() -> (w196:dbl)  [unwired: 1 in]
        "Check" <- w196
        n143 = case shown="True" w195 {
          tunnel: w196 -> [w433 w435]
          tunnel: [w433 w436] -> w194
          frame False {
          }
          frame True {
            n144 = local write "Drehzahl SW"(1000.0) -> ()
            n145 = Multiply(x=w435, y=sgl 0.0) -> (x*y=w436:dbl)
          }
        }
        n146 = Select(t=0.0, s=w195, f="Drehzahl SW") -> (s? t:f=w199:dbl)
        n147 = feedback-in #1(w199, w197) -> ()
        n148 = Equal?(x=w318, y=w314) -> (x = y?=→"warm":bool)
        n149 = Equal?(x=w315, y=w314) -> (x = y?=→"kalt":bool)
        n150 = Index Array(array=w133, index=13) -> (element=w135:dbl)
        n151 = Index Array(array=w108, index=22) -> (element=w107:dbl)
        n152 = case shown="True" "Boolean" {
          tunnel: w108 -> [_ w432]
          tunnel: w133 -> [_ w425]
          tunnel: [0.0 w418] -> w186
          tunnel: [0.0 w415] -> w175
          tunnel: w103 -> [_ w412]
          frame False {
          }
          frame True {
            n153 = Index Array(array=w412, index=8) -> (element=w414:dbl)
            n154 = Index Array(array=w425, index #1=4 ("index"), index #2=8 ("index")) -> (element #1=w420:dbl, element #2=w419:dbl)
            n155 = Index Array(array=w432, index #1=7 ("index"), index #2=6 ("index"), index #3=13 ("index"), index #4=14 ("index"), index #5=5 ("index")) -> (element #1=w424:dbl, element #2=w423:dbl, element #3=w422:dbl, element #4=w421:dbl, element #5=w416:dbl)
            n156 = script code="xi_a = xi_a/100;\ntry\nF = @(xi_r) ((refpropm('H','T',T6a+273.15,'P',p7*100,'ammonia','water',[xi_r 1-xi_r])*0.001-refpropm('H','T',T7+273.15,'P',p7*100,'ammonia','water',[xi_r 1-xi_r])*0.001)/(refpropm('H','T',T14+273.15,'P',p14*100,'ammonia','water',[xi_a 1-xi_a])*0.001-refpropm('H','T',T13+273.15,'P',p14*100,'ammonia','water',[xi_a 1-xi_a])*0.001)*(xi_a-1)+1-xi_r);\nxi_r0=xi_a;\n[xi_r, fval] = fzero(F,xi_r0);\n\n\ncatch\nxi_r=1\np_liq=refpropm('P','T',T6+273.15,'Q',0,'ammonia','water',[xi_r 1-xi_r])/100;\nend"("T7"=w424, "T6a"=w423, "T13"=w422, "T14"=w421, "xi_a"=w414, "p7"=w420, "p14"=w419, "T6"=w416) -> ("xi_r"=w418:dbl, "p_liq"=w415:dbl)  [unwired: 1 in, 1 out]
          }
        }
        "xi_r" <- w186
        "p_liq" <- w175
        n157 = call "Pumpensteuerung_PID.vi"("reinitialize? (F)"="reinitialize? (F)", "PID Regelung Pumpe"="PID Regelung Pumpe", "FI13 SW in l/min"="FI13 SW in l/min", "Prozessvariable"=w135, "Pumpensteuerung"="Pumpensteuerung") -> ("upper limit"=w181:dbl)  [unwired: 4 in, 2 out]
        n158 = call "Senkenregler_PID.vi"("Regelventil 36"="Regelventil 36", "Solltemp."="TI35 SW", "Regelventil 34"="Regelventil 34", "Regler Senke"="Regler Senke", "reinitialize?"="reinitialize?", "Numeric"=w107) -> ("upper limit 2"=w190:dbl, "upper limit"=w188:dbl)  [unwired: 6 in, 2 out]
        n159 = call "Filter7"("Signal"=w181) -> ("Filtered Signal"=w180:dynamicdata)  [unwired: 9 in, 1 out]
        "Mittelwert" <- w180
        n160 = case shown="True" "Mittelwert?" {
          tunnel: w181 -> [w408 _]
          tunnel: [w408 w409] -> w182
          tunnel: w180 -> [_ w409]
          frame False {
          }
          frame True {
          }
        }
        n161 = Greater Than 0?(x="RV 33") -> (x > 0?=w223:bool)
        n162 = Less Than 0?(x="RV 33") -> (x < 0?=w222:bool)
        n163 = Select(t=w358, s=w222, f=w359) -> (s? t:f=w356:i32)
        n164 = Select(t=w358, s=w223, f=w359) -> (s? t:f=w357:i32)
        n165 = call "Filter9"("Signal"=w175) -> ("Filtered Signal"=w173:dynamicdata)  [unwired: 9 in, 1 out]
        "p_liq_mittel" <- w173
        n166 = Greater?(x=w173, y=15.0) -> (0:w172:dynamicdata)
        n167 = case shown="False" w172 {
          tunnel: [w404 15.0 ("y")] -> w171
          tunnel: w172 -> [w404 _]
          frame False {
          }
          frame True {
          }
        }
        n168 = Add(x="zusätzlicher Druck", y=w171) -> (x+y=w170:dynamicdata)
        n169 = call "Hochdruckregler_PID.vi"("Regler Hochdruck"="Regler Hochdruck", "Dynamic Data"=w170, "Solldruck"="PI05 SW", "PI05"=w133, "Exp.V"="Exp.V", "reinitialize? (F) in"="reinitialize? (F) in") -> ("upper limit out"=w110:dbl)  [unwired: 7 in, 2 out]
        n170 = call "Filter8"("Signal"=w110) -> ("Filtered Signal"=w177:dynamicdata)  [unwired: 9 in, 1 out]
        "Mittelwert 2" <- w177
        n171 = case shown="True" "Mittelwert 2" {
          tunnel: w110 -> [w406 _]
          tunnel: [w406 w407] -> w178
          tunnel: w177 -> [_ w407]
          frame False {
          }
          frame True {
          }
        }
        n172 = call "Stellungen_Namen2.vi"("Kühlventil"=w190, "Pumpensteuerung"=w182, "Regelventil 39"="Regelventil 39", "Exp.V"=w178, "Regelventil 14"=w188, "Meter"=w194, "zu"="zu", "auf"="auf", "Regelventil 35"="Regelventil 35") -> ("Dynamic Data"=w254:dynamicdata)  [unwired: 2 in]
        n173 = Merge Signals(w254, w357, w356) -> (w111:dynamicdata)
        n174 = call-poly "DAQmx Write (Multi-Chan Multi-Samp 1D Wfm).vi"("task/channels in"=w113, "auto start"=w114, "data"=w111, "error in"=w112) -> ()  [unwired: 9 in, 3 out]
        n175 = Build Array("PI05 SW", "TI35 SW", "FI13 SW in l/min") -> (w101:dbl[])
        n176 = Insert Into Array(array=w103, new element=w101) -> (w102:dbl[])  [unwired: 1 in]
        n177 = Index Array(array=w102, index=0) -> (element=w167:dbl)
        n178 = Index Array(array=w108, index=18) -> (element=w246:dbl)
        n179 = Index Array(array=w133, index #1=1, index #2=5, index #3=7, index #4=6) -> (element #1=w243:dbl, element #2=w242:dbl, element #3=w241:dbl, element #4=w240:dbl)
        n180 = Not Equal To 0?(x=w167) -> (x != 0?=w168:bool)
        n181 = call "Verdichternamen.vi"("Array"=w102) -> ("Dynamic Data"=w365:dynamicdata)  [unwired: 10 in]
        n182 = Divide(x=w243, y=w242) -> (x/y=w364:dbl)
        "Druckverhältnis" <- w364
        n183 = Subtract(x=w241, y=w240) -> (x-y=w376:dbl)
        n184 = Greater?(x=w376, y=1.0) -> (0:w248:bool)
        "Fl.Pumpe an" <- w248
        n185 = Less?(x=w246, y=60) -> (x < y?=w310:bool)
        "Temperatur Öl" <- w310
        n186 = Greater?(x=w364, y=1.5) -> (0:w362:bool)
        n187 = Not(x=w168) -> (.not. x?=w384:bool)
        n188 = Build Array(w310, w362) -> (→"Warnungen":bool[])
        n189 = call "Elapsed Time1"("Reset"=w384) -> ("Elapsed Time (s)"=w368:dbl)  [unwired: 11 in, 7 out]
        n190 = expression code="x-3600"(w368) -> (w367:dbl)
        n191 = call "Elapsed Time3"("Reset"="?") -> ("Elapsed Time (s)"=w370:dbl)  [unwired: 11 in, 7 out]
        n192 = Greater?(x=w368, y=720.0) -> (0:w249:bool)
        "Magnetventil" <- w249
        n193 = Build Array(w168, w249, w248) -> (→"Status Komponenten":bool[])
        n194 = expression code="x-3600"(w370) -> (w371:dbl)
        n195 = Seconds To Date/Time(time stamp (now)=w367) -> (date time rec=w311:T15)  [unwired: 1 in]
        n196 = Seconds To Date/Time(time stamp (now)=w371) -> (date time rec=w380:T15)  [unwired: 1 in]
        n197 = Unbundle By Name(w311) -> ("second"=w382:i32, "minute"=w381:i32, "hour"=w369:i32)
        n198 = Unbundle By Name(w380) -> ("second"=w379:i32, "minute"=w378:i32, "hour"=w372:i32)
        n199 = Bundle("second"=w382, "minute"=w381, "hour"=w369) -> (→"Verdichteraktivität":cluster{"second":i32, "minute":i32, "hour":i32})  [unwired: 1 in]
        n200 = Bundle("second"=w379, "minute"=w378, "hour"=w372) -> (→"Betriebszeit":cluster{"second":i32, "minute":i32, "hour":i32})  [unwired: 1 in]
        n201 = Merge Signals(w128, w127, w254, w365) -> (w273:dynamicdata)
        n202 = flat-sequence {
          tunnel: [w465] -> w392
          tunnel: [w464] -> w391
          tunnel: w291 -> [w463]
          tunnel: w290 -> [w462]
          tunnel: [w460] -> w287
          tunnel: "Identität" -> [w459]
          tunnel: "Dateiname" -> [w458]
          tunnel: "Speichern" -> [w457]
          tunnel: "tag" -> [w456]
          tunnel: w392 -> [w563]
          tunnel: w391 -> [w562]
          tunnel: [w558] -> w294
          tunnel: [w560] -> w293
          tunnel: w292 -> [w559]
          frame #0 {
            n203 = Index Array(array=w462) -> (element=w461:timestamp)  [unwired: 1 in]
            n204 = event shown="[1] \"Speichern\": Value Change" {
              selector: _ -> [_ _ _]
              dyn-events: _ -> [_ _ _]
              timeout: 5 -> [_ _ _]
              tunnel: [_ w475 _] -> w465
              tunnel: w463 -> [_ w470 _]
              tunnel: ["" w474 ""] -> w464
              tunnel: w461 -> [_ w473 w544]
              tunnel: [_ _ w542] -> w460
              tunnel: w459 -> [_ w472 _]
              tunnel: w458 -> [_ w471 _]
              tunnel: w457 -> [_ w469 _]
              tunnel: w456 -> [_ w468 _]
              event Timeout {
                n205 = event-data() -> ()  [unwired: 1 in, 1 out]
              }
              event "Speichern": Value Change {
                n206 = event-data() -> ()  [unwired: 1 in, 1 out]
                n207 = case shown="True" w469 {
                  tunnel: [w507 _] -> w475
                  tunnel: [w502 _] -> w474
                  tunnel: w473 -> [w494 _]
                  tunnel: w472 -> [w478 _]
                  tunnel: w471 -> [w490 _]
                  tunnel: w470 -> [w489 _]
                  tunnel: w468 -> [w477 _]
                  frame False {
                    w481 = "\r"
                    n208 = property on="Dateiname" class="Str"("DisabledEnum"=T4."Disabled and Grayed Out" ("Disabled")) -> ()  [unwired: 2 in, 2 out]
                    n209 = for {
                      N: 1 -> [_]
                      tunnel: ["Zeit"] -> w487 mode=indexing
                      tunnel: ["Kommentar"] -> w483 mode=indexing
                    }
                    n210 = Format Date/Time String(time format string (%c)="%d-%m-%Y_%H.%M ", seconds (now)=w494) -> (date/time string=w495:string)  [unwired: 1 in]
                    n211 = Concatenate Strings(w478, "\\", w495, w490, ".lvm" ("string")) -> (w497:string)
                    n212 = Insert Into Array(array=w489, index (row)=0, new element=w487) -> (w485:string[][])  [unwired: 1 in]
                    n213 = Build Path(base path=path "\\\\pcift88\\Studenten/HT-Waermepumpe/Messdaten" ("file path (dialog if empty)"), name or relative path=w497) -> (appended path=w492:path)
                    n214 = Concatenate Strings(w478, "\t", "tag: " ("string"), w477) -> (w476:string)
                    n215 = Insert Into Array(array=w485, new element=w483) -> (w484:string[][])  [unwired: 2 in]
                    n216 = Open/Create/Replace File(file path (use dialog)=w492, operation (0:open)=T11."replace or create with confirmation") -> (refnum out=→"refnum out":refnum<file>, error out=w507:errorcluster)  [unwired: 4 in, 1 out]
                    n217 = Transpose 2D Array(2D array=w484) -> (transposed array=w505:string[][])
                    n218 = Format Date/Time String(seconds (now)=w494) -> (date/time string=w504:string)  [unwired: 2 in]
                    n219 = Strip Path(path=w492) -> (name=w491:string)  [unwired: 1 out]
                    n220 = Array To Spreadsheet String(array=w505, 3:"%s" ("format string")) -> (spreadsheet string=w503:string)  [unwired: 1 in]
                    n221 = Concatenate Strings(w476, w481, w481, w491, w481, w481, w504, w481, w481, w503, w481, w481) -> (w502:string)
                  }
                  frame True {
                    n222 = local read "refnum out"() -> (w511:refnum<file>)
                    n223 = property on="Dateiname" class="Str"("DisabledEnum"=T4."Enabled" ("Disabled")) -> ()  [unwired: 2 in, 2 out]
                    n224 = Close File(refnum=w511) -> ()  [unwired: 1 in, 2 out]
                  }
                }
              }
              event "Comment": Value Change {
                # "Umlaute + ß ersetzen, quick&dirty 4.1.2016"
                n225 = event-data() -> ()  [unwired: 1 in, 1 out]
                n226 = flat-sequence {
                  tunnel: ["Kommentar"] -> w512
                  tunnel: w544 -> [w548]
                  frame #0 {
                    w550 = "\r"
                    n227 = local read "Historie"() -> (w552:string)
                    n228 = Get Date/Time String(seconds (now)=w548, want seconds? (F)=TRUE) -> (time string=w551:string)  [unwired: 1 in, 1 out]
                    n229 = Concatenate Strings(w552, w551, " -> ", "Kommentar", w550, w550) -> (→"Historie":string)
                  }
                  frame #1 {
                    n230 = local write "Kommentar"("") -> ()
                  }
                }
                n231 = Search and Replace String(replace all?=TRUE, input string=w512, search string="ä", replace string="ae") -> (result string=w534:string)  [unwired: 4 in, 3 out]
                n232 = Search and Replace String(replace all?=TRUE, input string=w534, search string="ü", replace string="ue") -> (result string=w533:string)  [unwired: 4 in, 3 out]
                n233 = Search and Replace String(replace all?=TRUE, input string=w533, search string="ö", replace string="oe") -> (result string=w532:string)  [unwired: 4 in, 3 out]
                n234 = Search and Replace String(replace all?=TRUE, input string=w532, search string="ß", replace string="ss") -> (result string=w513:string)  [unwired: 4 in, 3 out]
                n235 = Search and Replace String(replace all?=TRUE, input string=w513, search string="Ä", replace string="Ae") -> (result string=w522:string)  [unwired: 4 in, 3 out]
                n236 = Search and Replace String(replace all?=TRUE, input string=w522, search string="Ü", replace string="Ue") -> (result string=w521:string)  [unwired: 4 in, 3 out]
                n237 = Search and Replace String(replace all?=TRUE, input string=w521, search string="Ö", replace string="Oe") -> (result string=w514:string)  [unwired: 4 in, 3 out]
                n238 = for {
                  N: 1 -> [_]
                  tunnel: [w545] -> w542 mode=indexing
                  tunnel: w514 -> [w545]
                }
              }
            }
          }
          frame #1 {
            n239 = local read "refnum out"() -> (w555:refnum<file>)
            n240 = Concatenate Strings(w562, w559) -> (w561:string)
            n241 = Not A Number/Path/Refnum?(number/path/refnum=w555) -> (NaN/Path/Refnum?=w556:bool)
            n242 = Set File Position(refnum=w555, from (0:start)=enum16{"start", "end", "current"}."end", error in=w563) -> (refnum out=w564:refnum<file>, error out=w565:errorcluster)  [unwired: 1 in]
            n243 = Not(x=w556) -> (.not. x?=→"Speichert!":bool)
            n244 = Write to Text File(file (use dialog)=w564, text=w561, error in=w565) -> (refnum out=w558:refnum<file>, error out=w560:errorcluster)  [unwired: 1 in, 1 out]
          }
        }
        n245 = Empty String/Path?(string/path="Identität") -> (empty?=w285:bool)
        n246 = Empty String/Path?(string/path="Dateiname") -> (empty?=w284:bool)
        n247 = Or(x=w285, y=w284) -> (x .or. y?=w281:bool)
        n248 = call "Protokollordnung"("Signals"=w273) -> ("Signal Out"=w299:dynamicdata)  [unwired: 9 in, 1 out]
        n249 = Boolean To (0,1)(Boolean=w281) -> (0, 1=w282:i16)
        n250 = expression code="x*2"(w282) -> (w283:i16)
        n251 = property on="Speichern" class="Bool (strict)"("DisabledEnum"=w283) -> ()  [unwired: 2 in, 2 out]
        n252 = call "Convert from Dynamic Data"("Dynamic Data Type"=w299) -> ("Array of Waveform"=w300:waveform(dbl)[])  [unwired: 3 in]
        n253 = Array Size(array=w300) -> (size(s)=w277:i32)
        n254 = Concatenate Strings("%" ("string"), "." ("string"), ";%g" ("string")) -> (w302:string)
        n255 = Initialize Array(w302, w277) -> (w301:string[])
        n256 = for {
          tunnel: w300 -> [w569] mode=indexing
          tunnel: [w576] -> w297 mode=indexing
          tunnel: w301 -> [w574] mode=indexing
          tunnel: [w568] -> w291 mode=indexing
          tunnel: [w570] -> w290 mode=indexing
          tunnel: [w571] -> w296 mode=indexing
          n257 = Unbundle By Name(w569) -> ("Y"=w575:dbl[], "t0"=w567:timestamp)
          n258 = Get Waveform Attribute(5:w567, 6:"NI_ExpTimeStamp", 7:w569) -> (1:w570:timestamp)  [unwired: 1 in, 3 out]
          n259 = for {
            tunnel: w575 -> [w583] mode=indexing
            tunnel: [w582] -> w576 mode=indexing
            tunnel: w574 -> [w581]
            tunnel: w569 -> [w580]
            tunnel: [w579] -> w568 mode=indexing
            n260 = Format Into String(format string=w581, w583) -> (resulting string=w582:string)  [unwired: 2 in, 1 out]
            n261 = Get Waveform Attribute(5:"", 6:"NI_ChannelName", 7:w580) -> (1:w579:string)  [unwired: 1 in, 3 out]
          }
          n262 = Format Date/Time String(time format string (%c)="%H.%M.%S", seconds (now)=w570) -> (date/time string=w571:string)  [unwired: 1 in]
        }
        n263 = Insert Into Array(array=w297, index (row)=0, new element=w296) -> (w288:string[][])  [unwired: 1 in]
        n264 = Increment(x=w277) -> (x+1=w278:i32)
        n265 = Insert Into Array(array=w288, index (row)=w278, new element=w287) -> (w289:string[][])  [unwired: 1 in]
        n266 = Transpose 2D Array(2D array=w289) -> (transposed array=w286:string[][])
        n267 = Array To Spreadsheet String(array=w286, 3:"%s" ("format string")) -> (spreadsheet string=w292:string)  [unwired: 1 in]
      }
      frame #2 {
        n268 = Tick Count (ms)() -> (millisecond timer value=w702:u32)
        n269 = Subtract(x=w702, y=w701) -> (x-y=w700:u32)
        n270 = Divide(x=w700, y=1000.0) -> (x/y=→"Schleifendauer":dbl)
      }
    }
  }
  n271 = call <vilib>:"DAQmx Clear Task.vi"("task in"=w6, "error in"=w4) -> ()  [unwired: 13 in, 1 out]
  n272 = call <vilib>:"DAQmx Clear Task.vi"("task in"=w5, "error in"=w3) -> ()  [unwired: 13 in, 1 out]
  n273 = Close File(refnum=w31, error in=w30) -> (error out=w34:errorcluster)  [unwired: 1 out]
  n274 = call <vilib>:"General Error Handler.vi"("error in (no error)"=w34, "[exception action] (none:0)"=1 ("[exception code]"), "[exception code]"=1) -> ()  [unwired: 8 in, 5 out]
